vi "Fetch Waveform.vi"(8 "error in (no error)":errorcluster, 9 "Timeout (10000 ms)":u32=10000, 10 "Channel (0: Channel 1)":u16(ring) items=["Channel 1", "Channel 2", "Channel 3", "Channel 4"], 11 "VISA resource name":refnum<visa-resource-name>) -> (0 "error out":errorcluster, 2 "Waveform Data":waveform(dbl)(graph), 3 "VISA resource name out":refnum<visa-resource-name>)   [LabVIEW 2012, in "RIGOL DS1000 Series.lvlib"]
doc: "Returns the waveform the oscilloscope acquired for the specified channel. The waveform is from an acquisition that you initiate prior to calling this VI.\n\n<B>Note:</B>\n Use this VI only with other low-level VIs."
uses:
  RIGOL DS1000 Series.lvlib
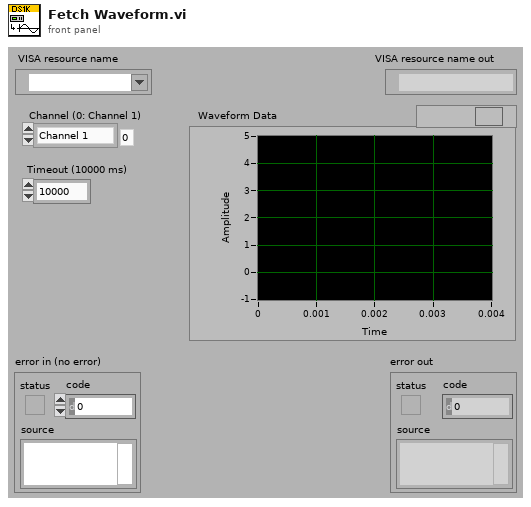
[diagram p1: front panel]
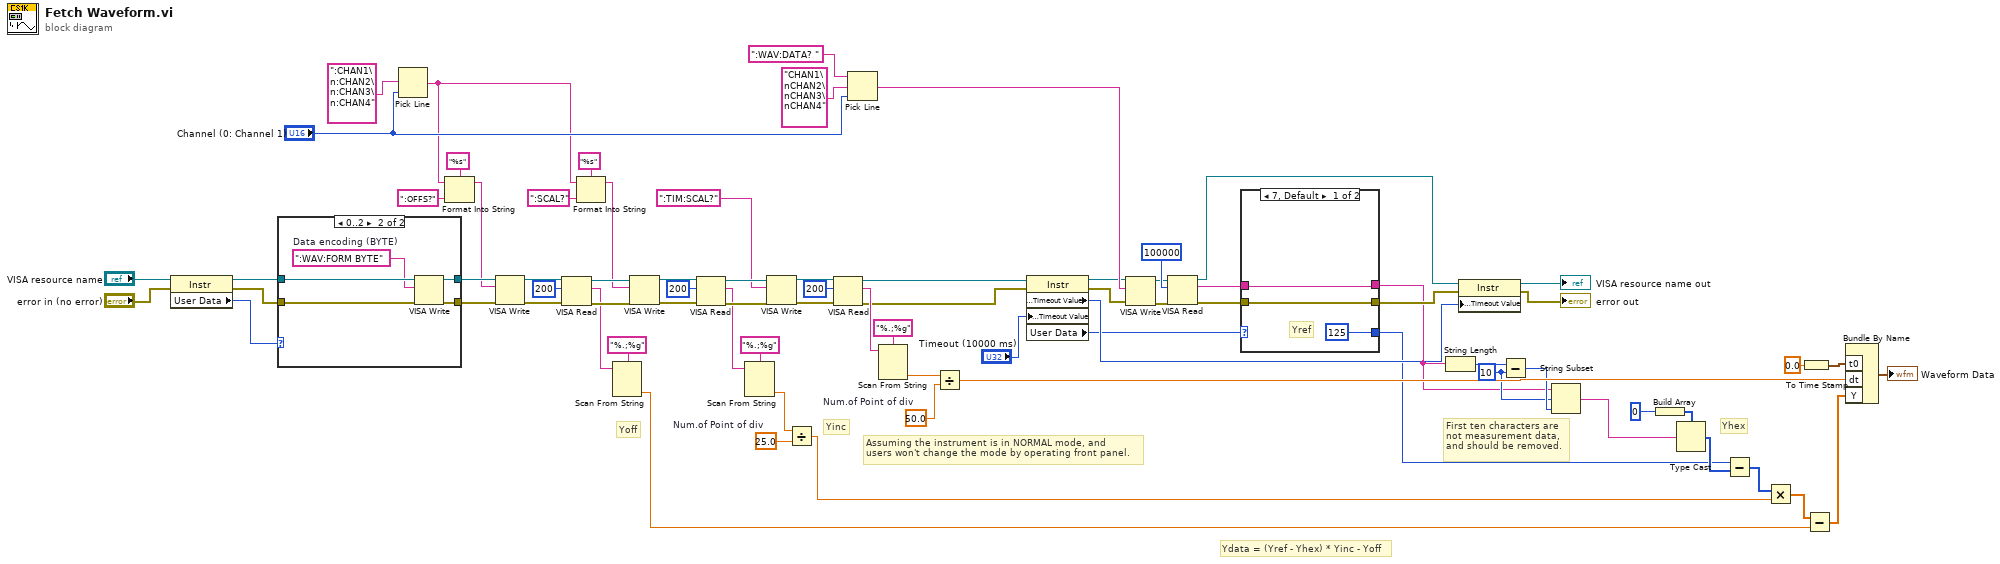
[diagram p0: block diagram]
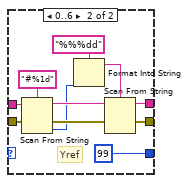
[diagram p2: hidden frame]
diagram:
  w3 = 10 ("y")
  w15 = 50.0  # Num.of Point of div
  w24 = 25.0  # Num.of Point of div
  # "Assuming the instrument is in NORMAL mode, and \nusers won't change the mode by operating front panel."
  # "First ten characters are\nnot measurement data, \nand should be removed."
  # "Yoff"
  # "Yinc"
  # "Yhex"
  # "Ydata = (Yref - Yhex) * Yinc - Yoff"
  n1 = property class="Instr"(reference="VISA resource name", error in="error in (no error)") -> (reference out=w56:refnum<visa-resource-name>, error out=w54:errorcluster, "User Data"=w33:u32)
  n2 = case shown="0..2" w33 {
    tunnel: [w79 w84] -> w52
    tunnel: [w78 w83] -> w51
    tunnel: w56 -> [w79 w82]
    tunnel: w54 -> [w78 w81]
    frame 3, Default {
    }
    frame 0..2 {
      w80 = ":WAV:FORM BYTE"  # Data encoding (BYTE)
      n3 = VISA Write(VISA resource name=w82, write buffer=w80, error in (no error)=w81) -> (VISA resource name out=w84:refnum<visa-resource-name>, error out=w83:errorcluster)  [unwired: 1 out]
    }
  }
  n4 = Pick Line(multi-line string=":CHAN1\n:CHAN2\n:CHAN3\n:CHAN4" ("多行字符串"), line index="Channel (0: Channel 1)") -> (output string=w34:string)  [unwired: 1 out]
  n5 = Format Into String(format string="%s" ("格式字符串"), initial string=w34, ":OFFS?") -> (resulting string=w30:string)  [unwired: 1 in, 1 out]
  n6 = VISA Write(VISA resource name=w52, write buffer=w30, error in (no error)=w51) -> (VISA resource name out=w50:refnum<visa-resource-name>, error out=w49:errorcluster)  [unwired: 1 out]
  n7 = VISA Read(VISA resource name=w50, byte count=u32 200, error in (no error)=w49) -> (VISA resource name out=w42:refnum<visa-resource-name>, read buffer=w32:string, error out=w41:errorcluster)  [unwired: 1 out]
  n8 = Format Into String(format string="%s" ("格式字符串"), initial string=w34, ":SCAL?") -> (resulting string=w29:string)  [unwired: 1 in, 1 out]
  n9 = Scan From String(format string="%.;%g", input string=w32) -> (output 1=w18:dbl)  [unwired: 2 in, 4 out]
  n10 = VISA Write(VISA resource name=w42, write buffer=w29, error in (no error)=w41) -> (VISA resource name out=w47:refnum<visa-resource-name>, error out=w48:errorcluster)  [unwired: 1 out]
  n11 = VISA Read(VISA resource name=w47, byte count=u32 200, error in (no error)=w48) -> (VISA resource name out=w38:refnum<visa-resource-name>, read buffer=w25:string, error out=w37:errorcluster)  [unwired: 1 out]
  n12 = Scan From String(format string="%.;%g", input string=w25) -> (output 1=w22:dbl)  [unwired: 2 in, 4 out]
  n13 = VISA Write(VISA resource name=w38, write buffer=":TIM:SCAL?", error in (no error)=w37) -> (VISA resource name out=w44:refnum<visa-resource-name>, error out=w43:errorcluster)  [unwired: 1 out]
  n14 = Divide(x=w22, y=w24) -> (x/y=w20:dbl)
  n15 = VISA Read(VISA resource name=w44, byte count=u32 200, error in (no error)=w43) -> (VISA resource name out=w8:refnum<visa-resource-name>, read buffer=w27:string, error out=w11:errorcluster)  [unwired: 1 out]
  n16 = Pick Line(string ("")=":WAV:DATA? " ("write buffer"), multi-line string="CHAN1\nCHAN2\nCHAN3\nCHAN4" ("多行字符串"), line index="Channel (0: Channel 1)") -> (output string=w59:string)
  n17 = Scan From String(format string="%.;%g", input string=w27) -> (output 1=w16:dbl)  [unwired: 2 in, 4 out]
  n18 = Divide(x=w16, y=w15) -> (x/y=w14:dbl)
  n19 = property class="Instr"(reference=w8, error in=w11, "General Settings:Timeout Value"="Timeout (10000 ms)") -> (reference out=w7:refnum<visa-resource-name>, error out=w10:errorcluster, "General Settings:Timeout Value"=w66:u32, "User Data"=w13:u32)
  n20 = VISA Write(VISA resource name=w7, write buffer=w59, error in (no error)=w10) -> (VISA resource name out=w6:refnum<visa-resource-name>, error out=w9:errorcluster)  [unwired: 1 out]
  n21 = VISA Read(VISA resource name=w6, byte count=u32 100000, error in (no error)=w9) -> (VISA resource name out=w70:refnum<visa-resource-name>, read buffer=w65:string, error out=w63:errorcluster)  [unwired: 1 out]
  n22 = case shown="7, Default" w13 {
    tunnel: [w87 w98] -> w2
    tunnel: [w86 w97] -> w69
    tunnel: w65 -> [w87 w90]
    tunnel: w63 -> [w86 w89]
    tunnel: [i16 125 ("t") i16 99 ("f")] -> w12
    frame 7, Default {
      # "Yref"
    }
    frame 0..6 {
      # "Yref"
      n23 = Scan From String(format string="#%1d", input string=w90, error in=w89) -> (remaining string=w94:string, error out=w92:errorcluster, output 1=w91:i32)  [unwired: 1 in, 2 out]
      n24 = Format Into String(format string="%%%dd", w91) -> (resulting string=w93:string)  [unwired: 2 in, 1 out]
      n25 = Scan From String(format string=w93, input string=w94, error in=w92) -> (remaining string=w98:string, error out=w97:errorcluster)  [unwired: 1 in, 3 out]
    }
  }
  n26 = String Length(string=w2) -> (length=w5:i32)
  n27 = property class="Instr"(reference=w70, error in=w69, "General Settings:Timeout Value"=w66) -> (reference out=→"VISA resource name out":refnum<visa-resource-name>, error out=→"error out":errorcluster)
  n28 = Subtract(x=w5, y=w3) -> (x-y=w4:i32)
  n29 = String Subset(string=w2, offset (0)=w3, length (rest)=w4) -> (substring=w1:string)
  n30 = Build Array(u8 0) -> (w74:u8[])
  n31 = Type Cast(type=w74, x=w1) -> (*(type *) &x=w23:u8[])
  n32 = Subtract(x=w12, y=w23) -> (x-y=w21:i16[])
  n33 = Multiply(x=w21, y=w20) -> (x*y=w19:dbl[])
  n34 = To Time Stamp(1:0.0 ("数字")) -> (0:w75:timestamp)
  n35 = Subtract(x=w19, y=w18) -> (x-y=w17:dbl[])
  n36 = Bundle By Name("t0"=w75, "dt"=w14, "Y"=w17) -> (→"Waveform Data":waveform(dbl))  [unwired: 1 out]
